vi "Version.vi"(0 "reference in":refnum<class "TestView_Tree.lvclass">, 11 "error in (no error)":errorcluster) -> (4 "reference in":refnum<class "TestView_Tree.lvclass">, 6 "Class":string, 8 "Chain":string, 10 "Version":string, 15 "error out":errorcluster)   [LabVIEW 2017]
uses:
  TestView_Tree.lvclass
  C:/Projects/Audinate/Src/Components/ViPER.lvlibp/ViPER.lvclass
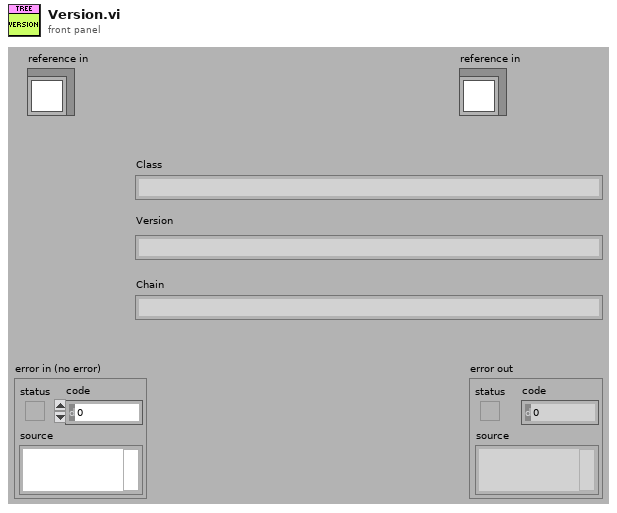
[diagram p1: front panel]
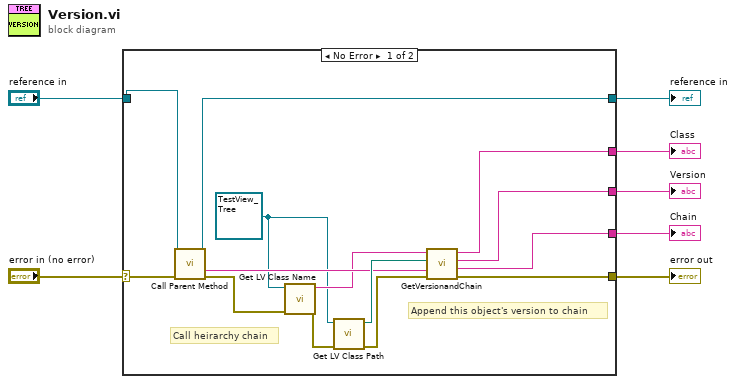
[diagram p0: block diagram]
diagram:
  n1 = case shown="No Error" "error in (no error)" {
    selector: "error in (no error)" -> [w19 w23]
    tunnel: [w15 w23] -> w4
    tunnel: [w20 w22] -> w7
    tunnel: "reference in" -> [w21 w22]
    tunnel: [w10 _] -> w3
    tunnel: [w12 _] -> w2
    tunnel: [w9 _] -> w1
    frame No Error {
      w8 = refnum<class "TestView_Tree.lvclass"> refnum ("reference in 2")
      # "Call heirarchy chain"
      # "Append this object's version to chain"
      n2 = call-parent "Call Parent Method"("reference in"=w21, "error in (no error)"=w19) -> ("reference out"=w20:refnum<class "TestView_Tree.lvclass">, "Chain"=w13:string, "error out"=w18:errorcluster)  [unwired: 9 in, 2 out]
      n3 = call <vilib>:"Get LV Class Name.vi"("error in (no error)"=w18, "object"=w8) -> ("error out"=w17:errorcluster, "class name"=w11:string)  [unwired: 8 in]
      n4 = call <vilib>:"Get LV Class Path.vi"("error in (no error)"=w17, "object"=w8) -> ("error out"=w16:errorcluster, "class path"=w14:path)  [unwired: 8 in]
      n5 = call "GetVersionandChain.vi"("error in (no error)"=w16, "Chain in"=w13, "class path in"=w14, "class name in"=w11) -> ("error out"=w15:errorcluster, "Chain out"=w9:string, "Version"=w12:string, "class name out"=w10:string)  [unwired: 4 in]
    }
    frame Error {
    }
  }
  "error out" <- w4
  "reference in" <- w7
  "Chain" <- w1
  "Version" <- w2
  "Class" <- w3
